vi "Preview State Bitfield.vi"(8 "error in (no error)":errorcluster, 11 "Valve in":refnum<class "Valve.lvclass">) -> (0 "error out":errorcluster, 2 "State Bitfield":u16, 3 "Valve out":refnum<class "Valve.lvclass">)   [LabVIEW 2015, in "cRIO-Carbondioxide.lvlib" / "CO2-Actor.lvlib" / "Valve.lvclass"]
uses:
  Valve.lvclass
  Valve.lvclass/Valve.ctl
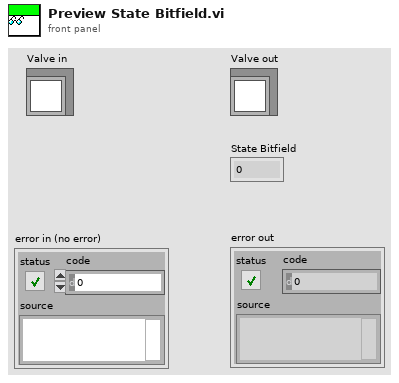
[diagram p1: front panel]
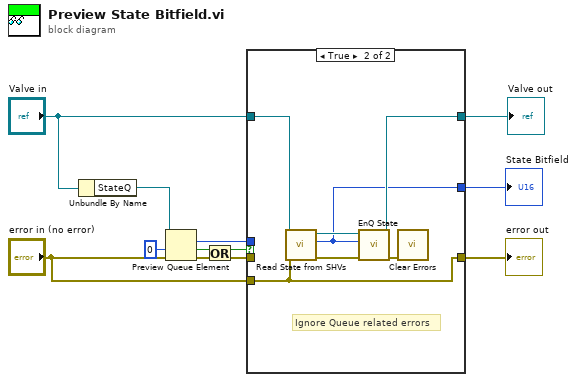
[diagram p0: block diagram]
diagram:
  n1 = Unbundle By Name("Valve in") -> ("StateQ"=w11:refnum<queue>)
  n2 = Preview Queue Element(queue=w11, timeout in ms (-1)=0, error in (no error)="error in (no error)") -> (element=w6:u16, timed out?=w4:bool, error out=w2:errorcluster)  [unwired: 1 out]
  n3 = Or(x=w4, y=w2) -> (x .or. y?=w3:bool)
  n4 = case shown="True" w3 {
    tunnel: w2 -> [w13 _]
    tunnel: [w13 w15] -> w9
    tunnel: "Valve in" -> [w14 w18]
    tunnel: [w14 w17] -> w7
    tunnel: w6 -> [w12 _]
    tunnel: [w12 w16] -> w5
    tunnel: "error in (no error)" -> [_ w15]
    frame False {
    }
    frame True {
      # "Ignore Queue related errors"
      n5 = call "Read State from SHVs.vi"("error in (no error)"=w15, "Valve in"=w18) -> ("error out"=w21:errorcluster, "BitField"=w16:u16, "Valve out"=w19:refnum<class "Valve.lvclass">)  [unwired: 7 in]
      n6 = call "EnQ State.vi"("error in (no error)"=w21, "BitField"=w16, "Valve in"=w19) -> ("error out"=w20:errorcluster, "Valve out"=w17:refnum<class "Valve.lvclass">)  [unwired: 7 in]
      n7 = call <vilib>:"Clear Errors.vi"("error in (no error)"=w20) -> ()  [unwired: 5 in, 2 out]
    }
  }
  "State Bitfield" <- w5
  "error out" <- w9
  "Valve out" <- w7
